vi "Generate Pure Mock Class.vi"(6 "Add to lvproj?":bool=TRUE, 8 "error in (no error)":errorcluster, 9 "Destination Class Path":path, 10 "Source Class Path":path) -> (0 "error out":errorcluster)   [LabVIEW 2020, in "Pure Mock Class Generator.lvclass"]
uses:
  Pure Mock Class Generator.lvclass
  Pure Mock Class Generator.lvclass/Pure Mock Class Generator.ctl
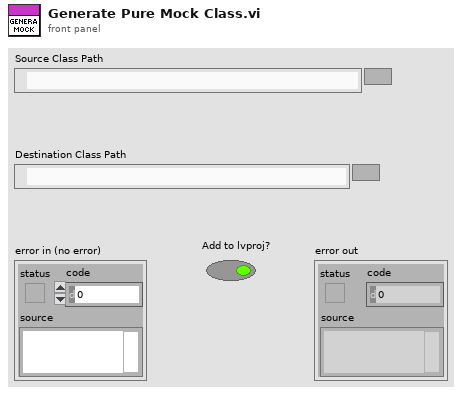
[diagram p1: front panel]
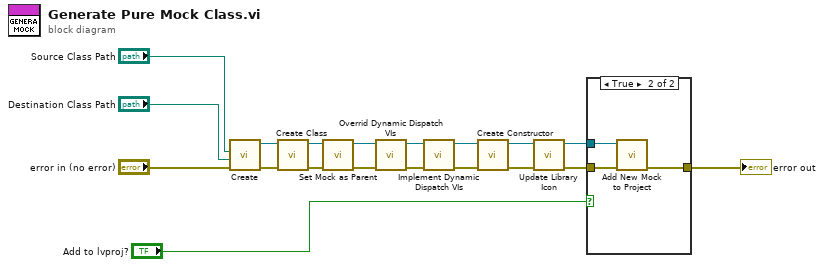
[diagram p0: block diagram]
diagram:
  n1 = call "Create.vi"("error in (no error)"="error in (no error)", "Destination Class Path"="Destination Class Path", "Source Class Path"="Source Class Path") -> ("error out"=w17:errorcluster, "Mock Class Generator Out"=w18:refnum<class "Pure Mock Class Generator.lvclass">)  [unwired: 7 in]
  n2 = call "Create Class.vi"("error in (no error)"=w17, "Mock Class Generator in"=w18) -> ("error out"=w7:errorcluster, "Mock Class Generator out"=w9:refnum<class "Pure Mock Class Generator.lvclass">)  [unwired: 8 in]
  n3 = call "Set Mock as Parent.vi"("error in (no error)"=w7, "Mock Class Generator in"=w9) -> ("error out"=w6:errorcluster, "Mock Class Generator out"=w8:refnum<class "Pure Mock Class Generator.lvclass">)  [unwired: 8 in]
  n4 = call "Overrid Dynamic Dispatch VIs.vi"("error in (no error)"=w6, "Mock Class Generator in"=w8) -> ("error out"=w13:errorcluster, "Mock Class Generator out"=w14:refnum<class "Pure Mock Class Generator.lvclass">)  [unwired: 8 in]
  n5 = call "Implement Dynamic Dispatch VIs.vi"("error in (no error)"=w13, "Mock Class Generator In"=w14) -> ("error out"=w12:errorcluster, "Mock Class Generator Out"=w10:refnum<class "Pure Mock Class Generator.lvclass">)  [unwired: 8 in]
  n6 = call "Create Constructor.vi"("error in (no error)"=w12, "Mock Class Generator in"=w10) -> ("error out"=w4:errorcluster, "Mock Class Generator"=w3:refnum<class "Pure Mock Class Generator.lvclass">)  [unwired: 8 in]
  n7 = call "Update Library Icon.vi"("error in (no error)"=w4, "Mock Class Generator In"=w3) -> ("error out"=w2:errorcluster, "Mock Class Generator Out"=w1:refnum<class "Pure Mock Class Generator.lvclass">)  [unwired: 8 in]
  n8 = case shown="True" "Add to lvproj?" {
    tunnel: w2 -> [w20 w23]
    tunnel: [w20 w22] -> w11
    tunnel: w1 -> [_ w21]
    frame False {
    }
    frame True {
      n9 = call "Add New Mock to Project.vi"("error in (no error)"=w23, "Mock Class Generator in"=w21) -> ("error out"=w22:errorcluster)  [unwired: 8 in, 1 out]
    }
  }
  "error out" <- w11
